vi "Set Icon Text Error Constant.vi"(8 "error in":errorcluster, 10 "Text":string, 11 "VI in":refnum<vi>) -> (0 "error out":errorcluster, 3 "VI out":refnum<vi>)   [LabVIEW 2020, in "ConstantErrorsMaker.lvlib"]
uses:
  ConstantErrorsMaker.lvlib
  <vilib>/LabVIEW Icon API/API_Text.ctl
  <vilib>/LabVIEW Icon API/API_User Layer Data.ctl
  <vilib>/Utility/miscctls.llb/LVPoint32TypeDef.ctl
  <vilib>/picture/picture.llb/imagedata.ctl
  <vilib>/LabVIEW Icon API/API_Test Settings.ctl
  <vilib>/LabVIEW Icon API/lv_icon/Controls/Alignment.ctl
  <vilib>/LabVIEW Icon API/API_Text Colors.ctl
  <vilib>/LabVIEW Icon API/LabVIEW Icon API.lvlib
  <vilib>/LabVIEW Icon API/lv_icon/lv_icon.lvlib
  <vilib>/LabVIEW Icon API/lv_icon/Controls/Pathes.ctl
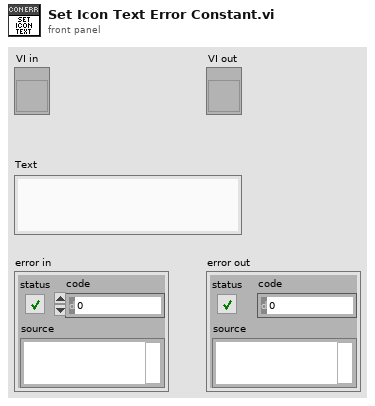
[diagram p1: front panel]
types:
  T1 = typedef "imagedata.ctl" = cluster{"image type":i32, "image depth":i32, "image":u8[], "mask":u8[], "colors":u32[], "Rectangle":cluster{"left":i16, "top":i16, "right":i16, "bottom":i16}}
  T2 = typedef "LabVIEW Icon API.lvlib/API_Test Settings.ctl" = cluster{"Font":string, "Alignment":T3, "Size":u8, "Center text":bool, "Capitalize text":bool, "Text color":T4}
  T3 = typedef "Alignment.ctl" = u16
  T4 = typedef "LabVIEW Icon API.lvlib/API_Text Colors.ctl" = cluster{"Line 1 color":u32, "Line 2 color":u32, "Line 3 color":u32, "Line 4 color":u32}
  T5 = typedef "LVPoint32TypeDef.ctl" = cluster{"Horizontal":i32, "Vertical":i32}
  T6 = typedef "LabVIEW Icon API.lvlib/API_User Layer Data.ctl" = cluster{"Layer name":string, "Origin":T5, "Icon image data":T1}
  T7 = typedef "LabVIEW Icon API.lvlib/API_Text.ctl" = cluster{"Line 1 text":string, "Line 2 text":string, "Line 3 text":string, "Line 4 text":string}
  T8 = typedef "Pathes.ctl" = enum16{"Root Path", "Icon Templates", "Icon Templates VI", "Icon Templates Lib", "Glyphs"}
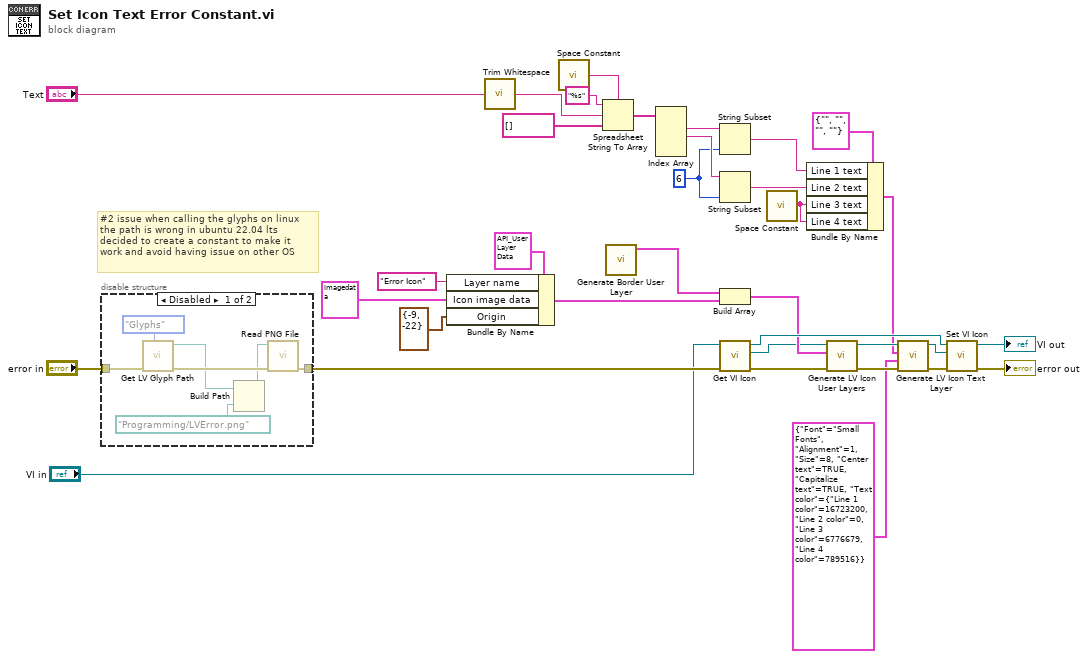
[diagram p0: block diagram]
diagram:
  w15 = 6 ("length (rest)")
  # "#2 issue when calling the glyphs on linux\nthe path is wrong in ubuntu 22.04 lts\ndecided to create a constant to make it \nwork and avoid having issue on other OS"
  n1 = disable-structure shown="Disabled" {
    disable-tunnel: "error in" -> [w41 w42]
    disable-tunnel: [w39 w42] -> w29
    frame Disabled {
      n2 = call <vilib>:"Get LV Glyph Path.vi"("Path"=Pathes."Glyphs", "error in (no error)"=w41) -> ("error out"=w40:errorcluster, "Requested Path"=w37:path)  [unwired: 1 in, 7 out]
      n3 = Build Path(base path=w37, name or relative path=path "Programming/LVError.png") -> (appended path=w36:path)
      n4 = call <vilib>:"Read PNG File.vi"("error in (no error)"=w40, "path to PNG file"=w36) -> ("error out"=w39:errorcluster)  [unwired: 7 in, 2 out]
    }
    frame Enabled {
    }
  }
  n5 = Bundle By Name(cluster=T6 {"Layer name"="", "Origin"={"Horizontal"=0, "Vertical"=0}, "Icon image data"={"image type"=0, "image depth"=0, "image"=[], "mask"=[], "colors"=[], "Rectangle"={"left"=0, "top"=0, "right"=0, "bottom"=0}}} ("User layer"), "Layer name"="Error Icon", "Icon image data"=T1 {"image type"=0, "image depth"=24, "image"=[255, 255, 255, 0, 0, 0, 0, 0, 0, 0, 0, 0, 0, 0, 0, 255, 255, 255, 255, 255, 255, 0, 0, 0, 0, 0, 0, 0, 0, 0, 0, 0, 0, 255, 255, 255, 255, 255, 255, 0, 0, 0, 0, 0, 0, 255, 255, 255, 0, 0, 0, 0, 0, 0, 0, 0, 0, 0, 0, 0, 255, 255, 255, 255, 255, 255, 0, 0, 0, 0, 0, 0, 255, 255, 255, 0, 0, 0, 0, 0, 0, 255, 255, 255, 255, 255, 255, 255, 255, 255, 255, 255, 255, 0, 0, 0, 0, 0, 0, 255, 255, 255, 0, 0, 0, 0, 0, 0, 255, 255, 255, 255, 255, 255, 0, 0, 0, 0, 0, 0, 255, 255, 255, 255, 255, 255, 255, 255, 255, 0, 0, 0, 0, 0, 0, 255, 255, 255, 255, 255, 255, 0, 0, 0, 0, 0, 0, 255, 255, 255, 255, 255, 255, 255, 255, 255, 0, 0, 0, 0, 0, 0, 255, 255, 255, 255, 255, 255, 255, 255, 255, 255, 255, 255, 255, 255, 255, 255, 255, 255, 255, 255, 255, 255, 255, 255, 255, 255, 255, 255, 255, 255, 255, 255, 255, 0, 0, 0, 0, 0, 0, 255, 255, 255, 255, 255, 255, 255, 255, 255, 0, 0, 0, 0, 0, 0, 255, 255, 255, 255, 255, 255, 0, 0, 0, 0, 0, 0, 255, 255, 255, 255, 255, 255, 255, 255, 255, 0, 0, 0, 0, 0, 0], "mask"=[], "colors"=[], "Rectangle"={"left"=0, "top"=0, "right"=9, "bottom"=9}} ("image data"), "Origin"=T5 {"Horizontal"=-9, "Vertical"=-22}) -> (w12:T6)
  n6 = call <vilib>:"Trim Whitespace.vi"("string"="Text") -> ("trimmed string"=w26:string)  [unwired: 1 in]
  n7 = call <vilib>:"Space Constant.vi"() -> ("String"=w24:string)
  n8 = Spreadsheet String To Array(delimiter (Tab)=w24, format string="%s", spreadsheet string=w26, array type (2D Dbl)=string[] [] ("format string")) -> (array=w22:string[])
  n9 = call <vilib>:"Generate Border User Layer.vi"() -> ("User Layer data"=w3:T6)  [unwired: 11 in]
  n10 = Index Array(array=w22) -> (element #1=w21:string, element #2=w20:string)  [unwired: 4 in, 2 out]
  n11 = String Subset(string=w21, length (rest)=w15) -> (substring=w19:string)  [unwired: 1 in]
  n12 = String Subset(string=w20, length (rest)=w15) -> (substring=w18:string)  [unwired: 1 in]
  n13 = Build Array(w3, w12) -> (w10:T6[])
  n14 = call <vilib>:"Get VI Icon.vi"("error in (no error)"=w29, "VI Refnum in"="VI in") -> ("error out"=w32:errorcluster, "Icon"=w7:refnum<class "Icon.lvclass">, "VI Refnum out"=w16:refnum<vi>)  [unwired: 7 in]
  n15 = call <vilib>:"Space Constant.vi"() -> ("String"=w2:string)
  n16 = Bundle By Name(cluster=T7 {"Line 1 text"="", "Line 2 text"="", "Line 3 text"="", "Line 4 text"=""} ("Text"), "Line 1 text"=w19, "Line 2 text"=w18, "Line 3 text"=w2, "Line 4 text"=w2) -> (w5:T7)
  n17 = call <vilib>:"Generate LV Icon User Layers.vi"("error in (no error)"=w32, "User layers"=w10, "Icon in"=w7) -> ("error out"=w31:errorcluster, "Icon out"=w8:refnum<class "Icon.lvclass">)  [unwired: 7 in]
  n18 = call <vilib>:"Generate LV Icon Text Layer.vi"("error in (no error)"=w31, "Text settings"=T2 {"Font"="Small Fonts", "Alignment"=1, "Size"=8, "Center text"=TRUE, "Capitalize text"=TRUE, "Text color"={"Line 1 color"=16723200, "Line 2 color"=0, "Line 3 color"=6776679, "Line 4 color"=789516}}, "Text"=w5, "Icon in"=w8) -> ("error out"=w30:errorcluster, "Icon out"=w6:refnum<class "Icon.lvclass">)  [unwired: 6 in]
  n19 = call <vilib>:"Set VI Icon.vi"("error in (no error)"=w30, "Icon"=w6, "VI Refnum in"=w16) -> ("error out"=→"error out":errorcluster, "VI Refnum out"=→"VI out":refnum<vi>)  [unwired: 7 in]
